vi "CC_G1st8_v2_sub.vi"(2 "macros2":i32[](array[numeric]), 3 "macros1":i32[](array[numeric])) -> (0 "Taus":dbl[](array[numeric]) format="%.2f", 1 "G1st8":dbl[](array[numeric])=[-0.39951995624066533, 0.3092433740982215, 0.20096008751866937, 0.1911161523750737, 0.07298893065192591, 0.20096008751866937, 0.20096008751866937, 0.013925319790352003] format="%.9f")   [LabVIEW 2009]
uses:
  <vilib>/Analysis/NI_AALPro.lvlib
panel:
  out "max(x,y)":i32
  out "x*y 2":i32[](graph)
  out "x*y":i32[](graph)
  out "x-y":i32[](graph)
  out "Numeric 3":i32
  out "Numeric 2":i32
  out "x+y":i32
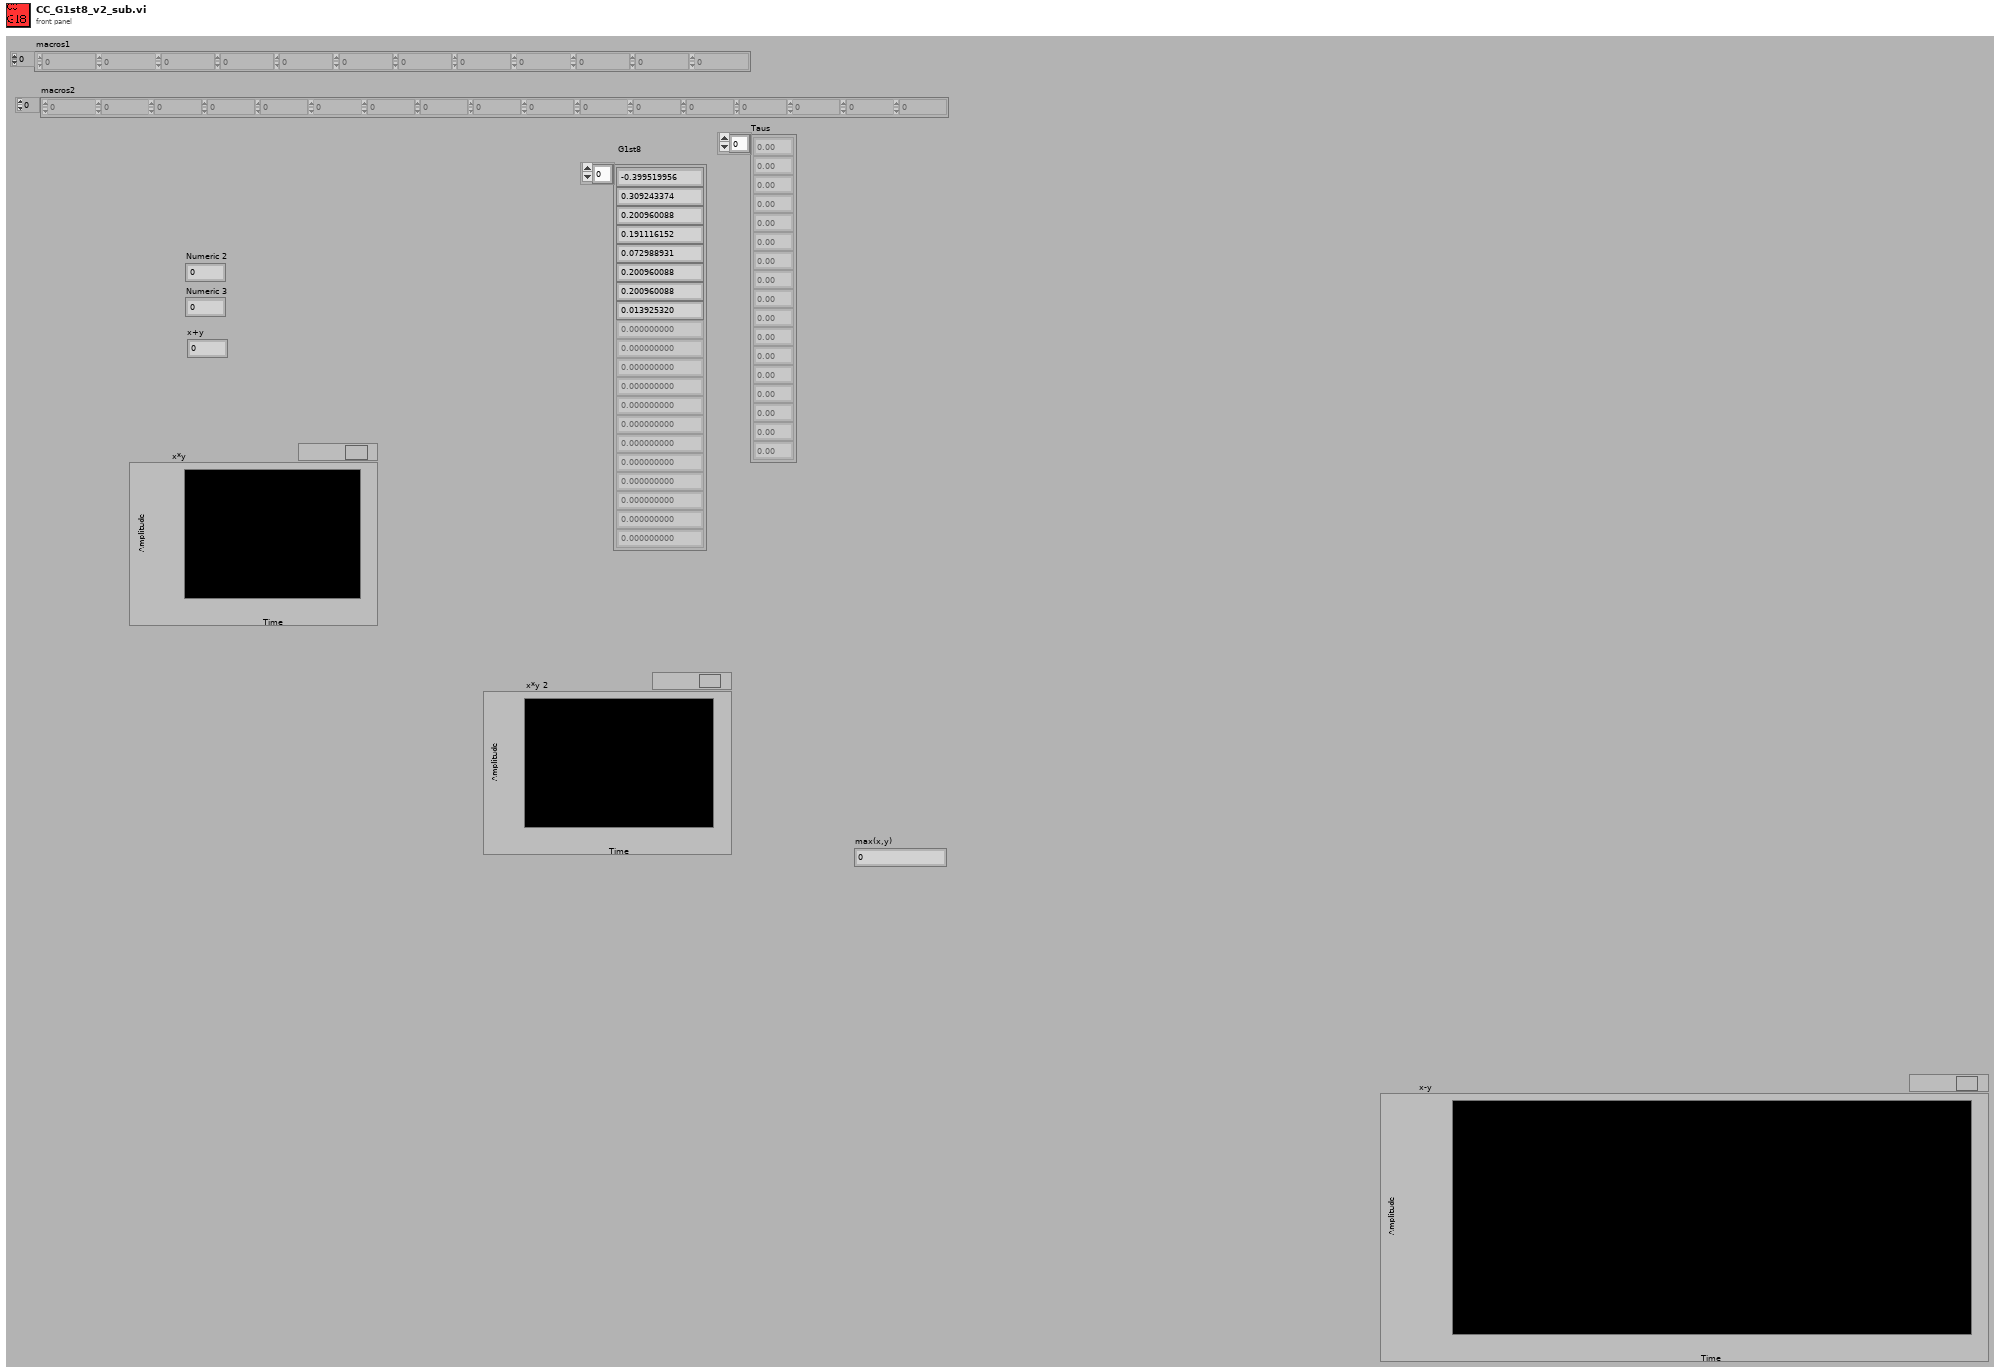
[diagram p1: front panel]
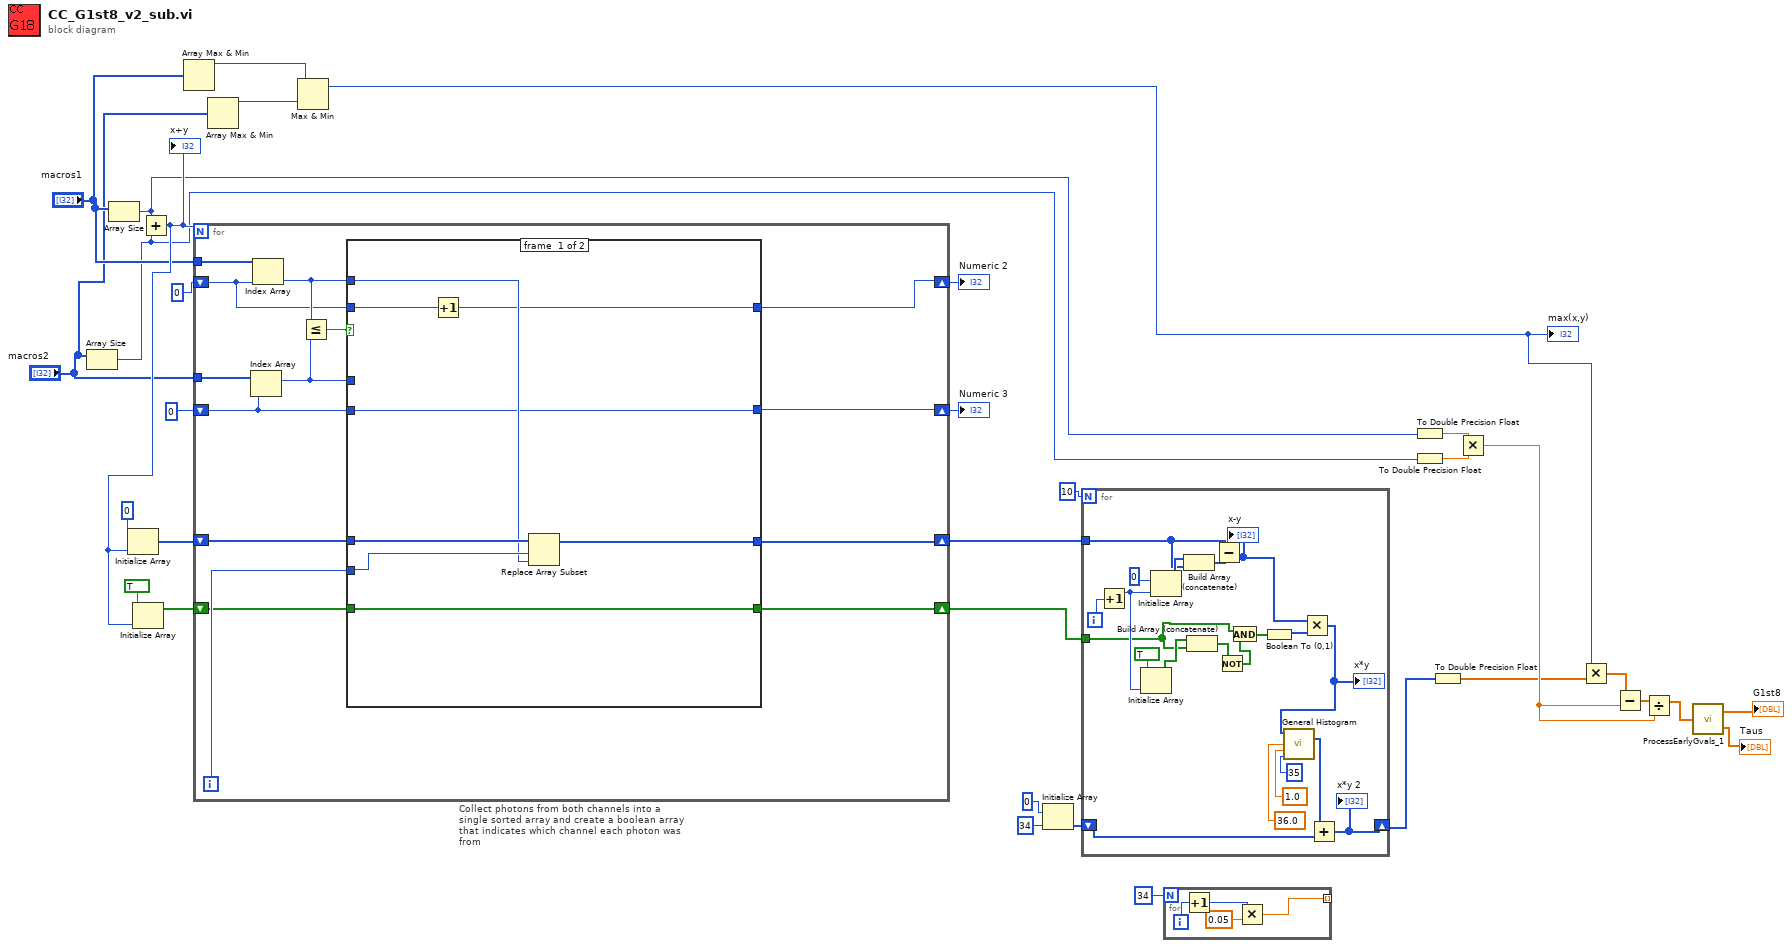
[diagram p0: block diagram]
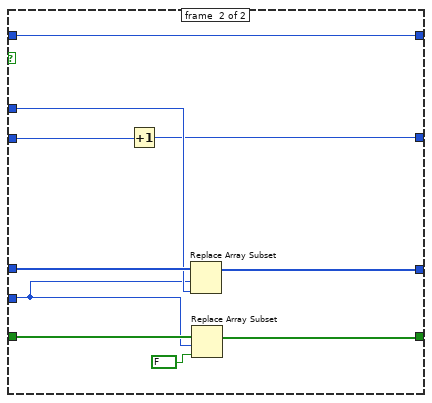
[diagram p2: hidden frame]
diagram:
  n1 = Array Size(array="macros2") -> (size(s)=w5:i32)
  n2 = Array Size(array="macros1") -> (size(s)=w6:i32)
  n3 = Add(x=w6, y=w5) -> (x+y=w25:i32)
  "x+y" <- w25
  n4 = Initialize Array(0, w25) -> (w30:i32[])
  n5 = Initialize Array(TRUE, w25) -> (w28:bool[])
  n6 = Array Max & Min(array="macros1") -> (max value=w22:i32)  [unwired: 3 out]
  n7 = for "Collect photons from both channels into a single sorted array and create a boolean array that indicates which channel each photon was from" {
    N: w25 -> [_]
    tunnel: "macros1" -> [w47]
    tunnel: "macros2" -> [w46]
    shift-right: [w36] -> w27
    shift-left: 0 -> [w37]
    shift-right: [w34] -> w26
    shift-left: 0 -> [w35]
    shift-right: [w38] -> w4
    shift-left: w30 -> [w44]
    shift-right: [w40] -> w10
    shift-left: w28 -> [w41]
    i -> [w43]
    n8 = Index Array(array=w46, index=w35) -> (element=w39:i32)
    n9 = Index Array(array=w47, index=w37) -> (element=w42:i32)
    n10 = Less Or Equal?(x=w42, y=w39) -> (x <= y?=w45:bool)
    n11 = case shown="False" w45 {
      tunnel: w44 -> [w55 w65]
      tunnel: w43 -> [w54 w61]
      tunnel: w42 -> [w53 _]
      tunnel: [w52 w64] -> w38
      tunnel: w41 -> [w51 w62]
      tunnel: [w51 w59] -> w40
      tunnel: w39 -> [_ w63]
      tunnel: w37 -> [w50 w58]
      tunnel: [w49 w58] -> w36
      tunnel: w35 -> [w48 w57]
      tunnel: [w48 w56] -> w34
      frame #0 {
        n12 = Increment(x=w50) -> (x+1=w49:i32)
        n13 = Replace Array Subset(array=w55, new element=w53, index=w54) -> (w52:i32[])
      }
      frame #1 {
        n14 = Increment(x=w57) -> (x+1=w56:i32)
        n15 = Replace Array Subset(array=w65, new element=w63, index=w61) -> (w64:i32[])
        n16 = Replace Array Subset(array=w62, new element=FALSE, index=w61) -> (w59:bool[])
      }
    }
  }
  "Numeric 2" <- w27
  "Numeric 3" <- w26
  n17 = Array Max & Min(array="macros2") -> (max value=w21:i32)  [unwired: 3 out]
  n18 = Max & Min(x=w22, y=w21) -> (max(x,y)=w9:i32)  [unwired: 1 out]
  "max(x,y)" <- w9
  n19 = Initialize Array(0 ("Element Data"), 34 ("Dimension Size")) -> (w18:i32[])
  n20 = for {
    N: 10 -> [_]
    tunnel: w4 -> [w83]
    shift-right: [w69] -> w12
    shift-left: w18 -> [w79]
    tunnel: w10 -> [w68]
    i -> [w77]
    n21 = Increment(x=w77) -> (x+1=w76:i32)
    n22 = Initialize Array(TRUE, w76) -> (w74:bool[])
    n23 = Initialize Array(0 ("Element Data"), w76) -> (w84:i32[])
    n24 = Build Array (concatenate)(w84, w83) -> (w86:i32[])
    n25 = Build Array (concatenate)(w74, w68) -> (w67:bool[])
    n26 = Subtract(x=w83, y=w86) -> (x-y=w71:i32[])
    "x-y" <- w71
    n27 = Not(x=w67) -> (.not. x?=w66:bool[])
    n28 = And(x=w68, y=w66) -> (x .and. y?=w73:bool[])
    n29 = Boolean To (0,1)(Boolean=w73) -> (0, 1=w72:i16[])
    n30 = Multiply(x=w71, y=w72) -> (x*y=w70:i32[])
    "x*y" <- w70
    n31 = call <vilib>:"General Histogram.vi"("X"=w70, "max"=36.0, "min"=1.0, "# bins"=35) -> ("Histogram"=w78:i32[])  [unwired: 7 in, 4 out]
    n32 = Add(x=w78, y=w79) -> (x+y=w69:i32[])
    "x*y 2" <- w69
  }
  n33 = for {
    N: 34 -> [_]
    tunnel: [w89] -> _ mode=indexing
    i -> [w88]
    n34 = Increment(x=w88) -> (x+1=w87:i32)
    n35 = Multiply(x=w87, y=0.05) -> (x*y=w89:dbl)
  }
  n36 = To Double Precision Float(number=w6) -> (double precision float=w8:dbl)
  n37 = To Double Precision Float(number=w5) -> (double precision float=w7:dbl)
  n38 = To Double Precision Float(number=w12) -> (double precision float=w11:dbl[])
  n39 = Multiply(x=w8, y=w7) -> (x*y=w15:dbl)
  n40 = Multiply(x=w9, y=w11) -> (x*y=w14:dbl[])
  n41 = Subtract(x=w14, y=w15) -> (x-y=w16:dbl[])
  n42 = Divide(x=w16, y=w15) -> (x/y=w3:dbl[])
  n43 = call "ProcessEarlyGvals_1.vi"("G2 vals in"=w3) -> ("G2 vals out"=→"G1st8":dbl[], "Tau Values"=→"Taus":dbl[])
